vi "SizeGraphPanelV2.vi"(8 "ErrorIn(No Error)":errorcluster caption="entrée d'erreur (pas d'erreur)", 9 "Width Divider":i32, 10 "Height Divider":i32, 11 "PanRef":refnum<vi>) -> (0 "sortie d'erreur":errorcluster, 2 "Position":T1, 3 "cluster de sortie":T2 caption="Taille")   [LabVIEW 2019]
uses:
  <vilib>/Utility/miscctls.llb/LVBoundsTypeDef.ctl
  <vilib>/Utility/miscctls.llb/LVPositionTypeDef.ctl
  <vilib>/Utility/miscctls.llb/LVPointTypeDef.ctl
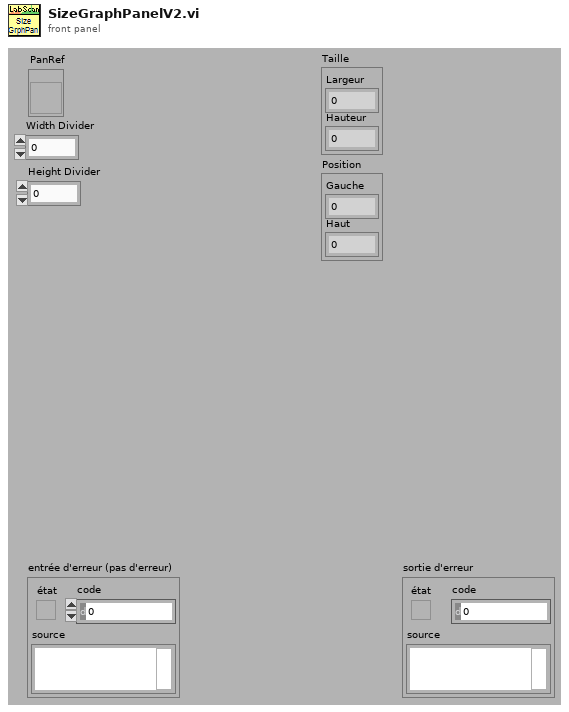
[diagram p1: front panel]
types:
  T1 = typedef "LVPositionTypeDef.ctl" = cluster{"Left":i32, "Top":i32}
  T2 = typedef "LVBoundsTypeDef.ctl" = cluster{"Width":u32, "Height":u32}
  T3 = enum16{"Always On", "Always Off", "Off While Running"}
  T4 = typedef "LVPointTypeDef.ctl" = cluster{"Horizontal":i16, "Vertical":i16}
  T5 = typedef "LVRectTypeDef.ctl" = cluster{"Left":i16, "Top":i16, "Right":i16, "Bottom":i16}
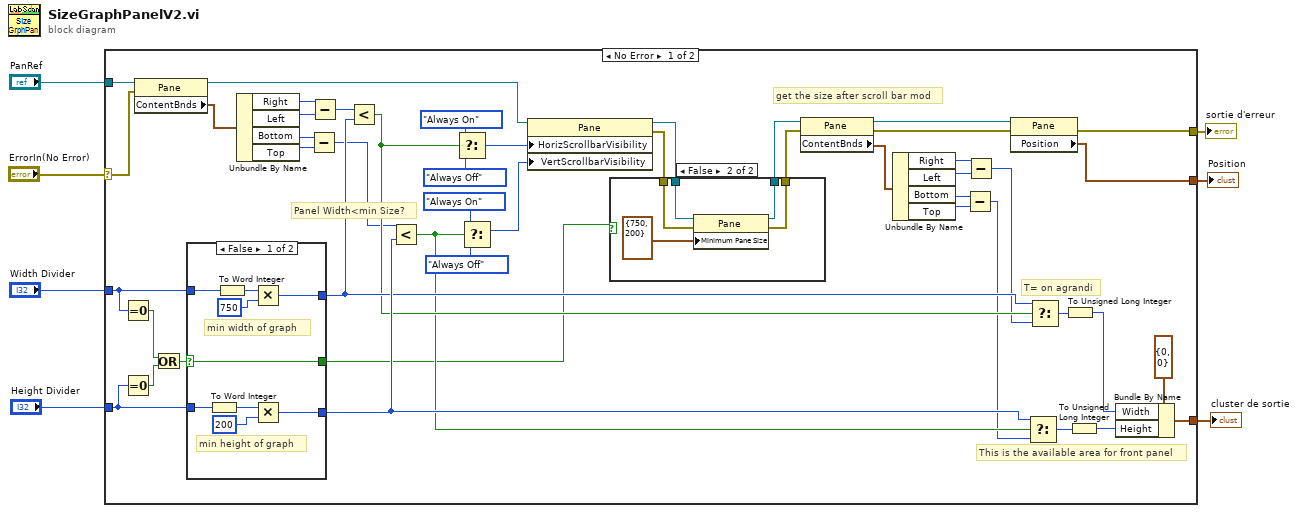
[diagram p0: block diagram]
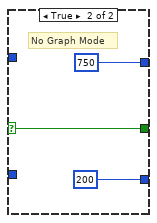
[diagram p2: hidden frame]
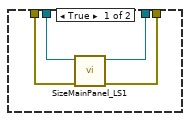
[diagram p3: hidden frame]
diagram:
  n1 = case shown="No Error" "ErrorIn(No Error)" {
    selector: "ErrorIn(No Error)" -> [w29 w76]
    tunnel: [w54 w76] -> w6
    tunnel: "PanRef" -> [w30 _]
    tunnel: "Width Divider" -> [w34 _]
    tunnel: "Height Divider" -> [w33 _]
    tunnel: [w47 _] -> w2
    tunnel: [w53 _] -> w1
    frame No Error {
      # "This is the available area for front panel"
      # "get the size after scroll bar mod"
      # "T= on agrandi"
      # "Panel Width<min Size?"
      n2 = Equal To 0?(x=w34) -> (x = 0?=w32:bool)
      n3 = Equal To 0?(x=w33) -> (x = 0?=w31:bool)
      n4 = property class="Pane"(reference=w30, error in=w29) -> (reference out=w40:refnum<vi>, "ContentBnds"=w35:T5)  [unwired: 1 out]
      n5 = Or(x=w32, y=w31) -> (x .or. y?=w9:bool)
      n6 = case shown="False" w9 {
        selector: w9 -> [w55 w64]
        tunnel: w34 -> [w59 _]
        tunnel: w33 -> [w58 _]
        tunnel: [w57 i16 200] -> w28
        tunnel: [w56 i16 750] -> w27
        tunnel: [w55 w64] -> w8
        frame False {
          # "min width of graph"
          # "min height of graph"
          n7 = To Word Integer(number=w58) -> (16bit integer=w60:i16)
          n8 = To Word Integer(number=w59) -> (16bit integer=w61:i16)
          n9 = Multiply(x=w61, y=i16 750) -> (x*y=w56:i16)
          n10 = Multiply(x=w60, y=i16 200) -> (x*y=w57:i16)
        }
        frame True {
          # "No Graph Mode"
        }
      }
      n11 = Unbundle By Name(w35) -> ("Right"=w36:i16, "Left"=w37:i16, "Bottom"=w39:i16, "Top"=w38:i16)
      n12 = Subtract(x=w39, y=w38) -> (x-y=w17:i16)
      n13 = Subtract(x=w36, y=w37) -> (x-y=w19:i16)
      n14 = Less?(x=w19, y=w27) -> (x < y?=w26:bool)
      n15 = Less?(x=w17, y=w28) -> (x < y?=w25:bool)
      n16 = Select(t=T3."Always On" ("Visibilité de la barre de défilement horizontale"), s=w26, f=T3."Always Off" ("Visibilité de la barre de défilement horizontale")) -> (s? t:f=w44:T3)
      n17 = Select(t=T3."Always On" ("Visibilité de la barre de défilement horizontale"), s=w25, f=T3."Always Off" ("Visibilité de la barre de défilement horizontale")) -> (s? t:f=w41:T3)
      n18 = property class="Pane"(reference=w40, "HorizScrollbarVisibility"=w44, "VertScrollbarVisibility"=w41) -> (reference out=w12:refnum<vi>, error out=w13:errorcluster)  [unwired: 1 in]
      n19 = case shown="False" w8 {
        tunnel: w13 -> [w68 w75]
        tunnel: w12 -> [w70 w74]
        tunnel: [w69 w73] -> w11
        tunnel: [w67 w72] -> w10
        frame True {
          n20 = call "SizeMainPanel_LS1.vi"("ErrorIn(No Error)"=w68, "PaneRef"=w70) -> ("sortie d'erreur"=w67:errorcluster, "PaneRef Out"=w69:refnum<vi>)  [unwired: 8 in]
        }
        frame False {
          n21 = property class="Pane"(reference=w74, error in=w75, "Minimum Pane Size"=T4 {"Horizontal"=750, "Vertical"=200} ("Taille minimale de panneau")) -> (reference out=w73:refnum<vi>, error out=w72:errorcluster)
        }
      }
      n22 = property class="Pane"(reference=w11, error in=w10) -> (reference out=w14:refnum<vi>, error out=w15:errorcluster, "ContentBnds"=w20:T5)
      n23 = Unbundle By Name(w20) -> ("Right"=w24:i16, "Left"=w23:i16, "Bottom"=w21:i16, "Top"=w22:i16)
      n24 = Subtract(x=w21, y=w22) -> (x-y=w16:i16)
      n25 = Subtract(x=w24, y=w23) -> (x-y=w18:i16)
      n26 = property class="Pane"(reference=w14, error in=w15) -> (error out=w54:errorcluster, "Position"=w47:T1)  [unwired: 1 out]
      n27 = Select(t=w28, s=w25, f=w16) -> (s? t:f=w52:i16)
      n28 = Select(t=w27, s=w26, f=w18) -> (s? t:f=w50:i16)
      n29 = To Unsigned Long Integer(number=w50) -> (unsigned 32bit integer=w49:u32)
      n30 = To Unsigned Long Integer(number=w52) -> (unsigned 32bit integer=w48:u32)
      n31 = Bundle By Name(cluster=T2 {"Width"=0, "Height"=0} ("cluster de sortie"), "Width"=w49, "Height"=w48) -> (w53:T2)
    }
    frame Error {
    }
  }
  "sortie d'erreur" <- w6
  "cluster de sortie" <- w1
  "Position" <- w2
